vi "Pre-Process.vi"(11 "TEMPLATE jettl in":refnum<class "TEMPLATE Actor.lvclass">) -> (3 "TEMPLATE jettl out":refnum<class "TEMPLATE Actor.lvclass">)   [LabVIEW 2021, in "_Template.lvlib" / "Templates.lvlib" / "TEMPLATE Actor.lvlib" / "TEMPLATE Actor.lvclass"]
uses:
  TEMPLATE Actor.lvclass
  jettl/jettl/Setup Msg/Setup Msg.lvlib
  jettl/jettl/Actor/Actor/Actor.lvclass
  jettl/jettl/Msg/Msg.lvclass
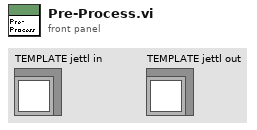
[diagram p1: front panel]
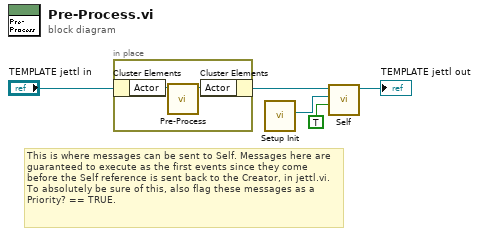
[diagram p0: block diagram]
diagram:
  # "This is where messages can be sent to Self. Messages here are guaranteed to execute as the first events since they come before the Self reference is sent back to the Creator, in jettl.vi. To absolutely be sure of this, also flag these messages as a Priority? == TRUE."
  n1 = in-place {
    n2 = in-place-cluster #1("TEMPLATE jettl in") -> ("Actor"=w7:refnum<class "Actor.lvclass">)
    n3 = call-dynamic "Pre-Process.vi"("Actor in"=w7) -> ("Actor out"=w6:refnum<class "Actor.lvclass">)  [unwired: 10 in]
    n4 = in-place-cluster #1("Actor"=w6) -> (w4:refnum<class "TEMPLATE Actor.lvclass">)
  }
  n5 = call "Setup Init.vi"() -> ("Msg"=w1:refnum<class "Msg.lvclass">)  [unwired: 11 in]
  n6 = call-dynamic "Self.vi"("Priority?"=TRUE, "Msg Strategy"=w1, "TEMPLATE jettl in"=w4) -> ("TEMPLATE jettl out"=→"TEMPLATE jettl out":refnum<class "TEMPLATE Actor.lvclass">)  [unwired: 8 in]
